vi "102KeyMappingPiano.vi"(11 "Double":dbl) -> (2 "signed 8bit integer":u8, 3 "Numeric":i8)   [LabVIEW 2016]
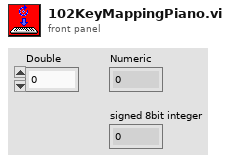
[diagram p1: front panel]
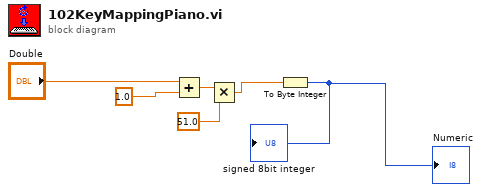
[diagram p0: block diagram]
diagram:
  n1 = Add(x="Double", y=1.0) -> (x+y=w2:dbl)
  n2 = Multiply(x=w2, y=51.0) -> (x*y=w4:dbl)
  n3 = To Byte Integer(number=w4) -> (8bit integer=→"signed 8bit integer" →"Numeric":i8)
